vi "Send Sync Pulse.vi"(8 "error in (no error)":errorcluster, 11 "VISA resource name":refnum<visa-resource-name>) -> (0 "error out":errorcluster, 3 "VISA resource name out":refnum<visa-resource-name>)   [LabVIEW 2014, in "Fluke 5XXX Series Multicalibrators.lvlib"]
doc: "This VI sends a synchronization pulse out to a slave Calibrator through the 10 MHZ OUT BNC connector.\n\nNote:\n\nThis VI is available only for instrument model 5520A."
uses:
  Fluke 5XXX Series Multicalibrators.lvlib
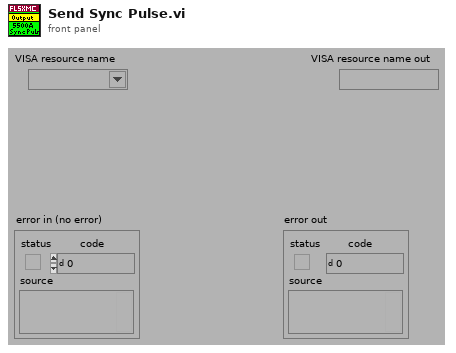
[diagram p1: front panel]
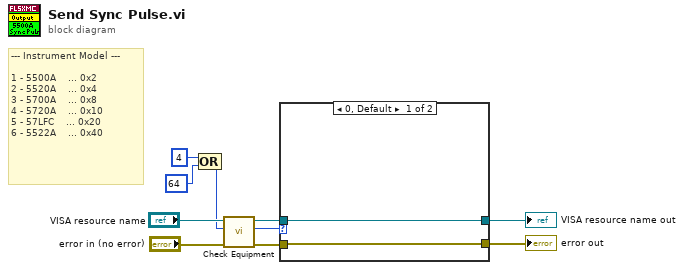
[diagram p0: block diagram]
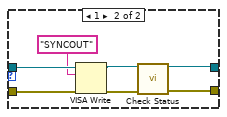
[diagram p2: hidden frame]
diagram:
  # "--- Instrument Model ---\n\n1 - 5500A    ... 0x2\n2 - 5520A    ... 0x4\n3 - 5700A    ... 0x8\n4 - 5720A    ... 0x10\n5 - 57LFC    ... 0x20\n6 - 5522A    ... 0x40"
  n1 = Compound Arithmetic op=OR(4 ("Numeric"), 64 ("Numeric")) -> (w1:i32)
  n2 = call "Check Equipment.vi"("error in (no error)"="error in (no error)", "Bit Mask"=w1, "VISA resource name"="VISA resource name") -> ("error out"=w10:errorcluster, "Present?"=w9:u32, "VISA resource name out"=w8:refnum<visa-resource-name>)  [unwired: 6 in]
  n3 = case shown="0, Default" w9 {
    tunnel: [w11 w14] -> w4
    tunnel: w10 -> [w12 w19]
    tunnel: w8 -> [w11 w18]
    tunnel: [w12 w17] -> w5
    frame 0, Default {
    }
    frame 1 {
      n4 = VISA Write(VISA resource name=w18, write buffer="SYNCOUT", error in (no error)=w19) -> (VISA resource name out=w15:refnum<visa-resource-name>, error out=w16:errorcluster)  [unwired: 1 out]
      n5 = call "Check Status.vi"("VISA resource name"=w15, "error in (no error)"=w16) -> ("VISA resource name out"=w14:refnum<visa-resource-name>, "error out"=w17:errorcluster)  [unwired: 12 in]
    }
  }
  "VISA resource name out" <- w4
  "error out" <- w5
